vi "test_Checksum U32 - Check Protection with corrupt data.vi"(8 "error in (no error)":errorcluster) -> (0 "error out":errorcluster)   [LabVIEW 2019, in "Protections Unit Tests.lvclass"]
uses:
  Protections Unit Tests.lvclass
  Checksum U32/Checksum U32.lvclass
  0c10e477-a100-4b93-935c-4b2bb0535a3f.vi
  <vilib>/addons/_JKI Toolkits/VI Tester/TestCase.llb/TestCase.lvclass
  C:/Program Files (x86)/National Instruments/LabVIEW 2019/vi.lib/addons/_JKI Toolkits/VI Tester/TestCase.llb/TestCase.lvclass
panel:
  out "Checksum U32 out":refnum<class "Checksum U32.lvclass">
  in  "Checksum U32 in":refnum<class "Checksum U32.lvclass">
  out "TestCase out":refnum<class "Protections Unit Tests.lvclass">
  in  "TestCase in":refnum<class "Protections Unit Tests.lvclass">
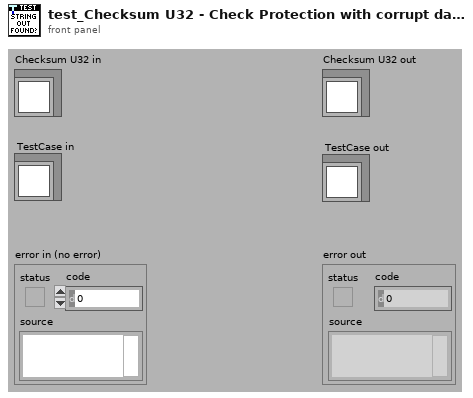
[diagram p1: front panel]
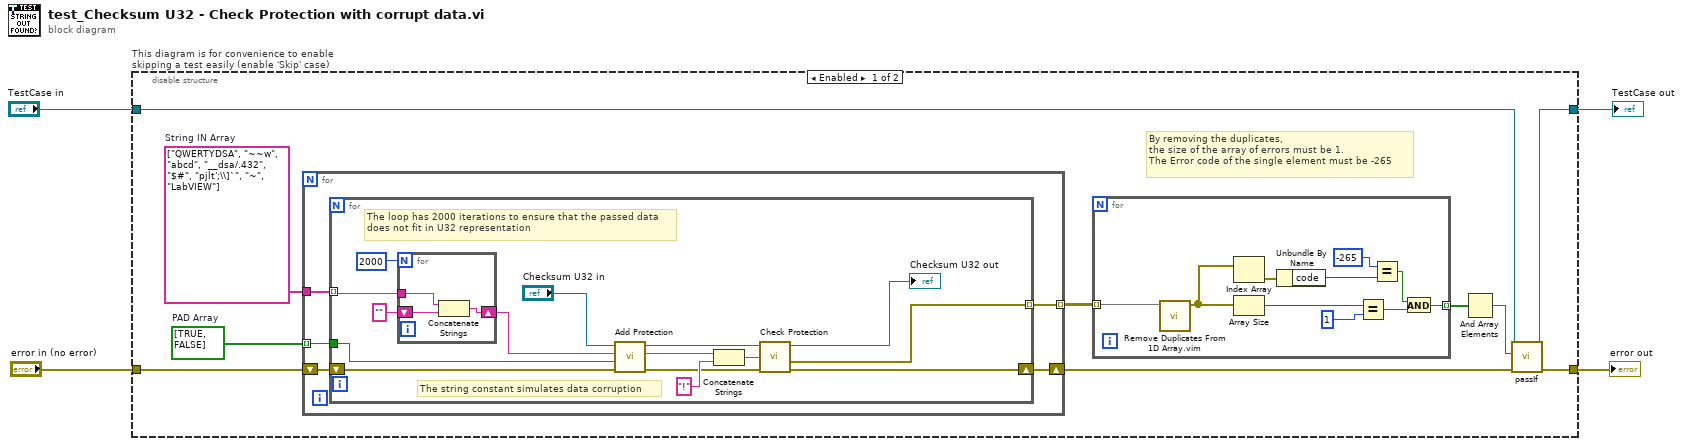
[diagram p0: block diagram]
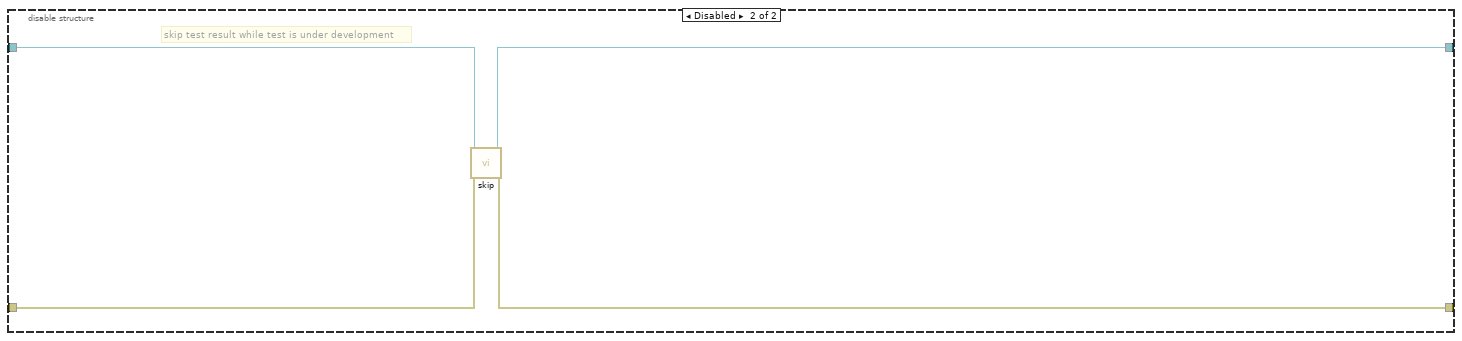
[diagram p2: hidden frame]
diagram:
  n1 = disable-structure "This diagram is for convenience to enable skipping a test easily (enable 'Skip' case)" shown="Enabled" {
    disable-tunnel: "TestCase in" -> [w12 w51]
    disable-tunnel: [w11 w49] -> w1
    disable-tunnel: [w10 w50] -> w3
    disable-tunnel: "error in (no error)" -> [w14 w48]
    frame Enabled {
      w5 = bool[] [TRUE, FALSE]  # PAD Array
      w13 = string[] ["QWERTYDSA", "~~w", "abcd", "__dsa/.432", "$#", "pjlt';\\]`", "~", "LabVIEW"]  # String IN Array
      # "By removing the duplicates, \nthe size of the array of errors must be 1. \nThe Error code of the single element must be -265"
      n2 = for {
        tunnel: w13 -> [w18]
        shift-right: [w17] -> w9
        shift-left: w14 -> [w19]
        tunnel: [w16] -> w6 mode=indexing
        tunnel: w5 -> [w15] mode=indexing
        n3 = for {
          tunnel: w18 -> [w32] mode=indexing
          shift-right: [w27] -> w17
          shift-left: w19 -> [w26]
          tunnel: [w28] -> w16 mode=indexing
          tunnel: w15 -> [w20]
          # "The string constant simulates data corruption"
          # "The loop has 2000 iterations to ensure that the passed data\ndoes not fit in U32 representation"
          n4 = for {
            N: 2000 -> [_]
            shift-right: [w37] -> w25
            shift-left: "" -> [w36]
            tunnel: w32 -> [w35]
            n5 = Concatenate Strings(w35, w36) -> (w37:string)
          }
          n6 = call-dynamic "Add Protection.vi"("error in (no error)"=w26, "Pad"=w20, "String in"=w25, "Checksum U32 in"="Checksum U32 in") -> ("error out"=w24:errorcluster, "String out"=w23:string, "Checksum U32 out"=w22:refnum<class "Checksum U32.lvclass">)  [unwired: 5 in]
          n7 = Concatenate Strings(w23, "!" ("string")) -> (w30:string)
          n8 = call-dynamic "Check Protection.vi"("error in (no error)"=w24, "String in"=w30, "Checksum U32 in"=w22) -> ("error out"=w27:errorcluster, "Protection Error"=w28:errorcluster, "Checksum U32 out"=→"Checksum U32 out":refnum<class "Checksum U32.lvclass">)  [unwired: 5 in, 1 out]
        }
      }
      n9 = for {
        tunnel: w6 -> [w47] mode=indexing
        tunnel: [w42] -> w8 mode=indexing
        n10 = call "Remove Duplicates From 1D Array.vim"("array"=w47) -> ("array with duplicates removed"=w43:errorcluster[])  [unwired: 10 in]
        n11 = Index Array(array=w43) -> (element=w39:errorcluster)  [unwired: 1 in]
        n12 = Array Size(array=w43) -> (size(s)=w38:i32)
        n13 = Unbundle By Name(w39) -> ("code"=w40:i32)
        n14 = Equal?(x=w38, y=1) -> (x = y?=w44:bool)
        n15 = Equal?(x=-265, y=w40) -> (x = y?=w45:bool)
        n16 = And(x=w45, y=w44) -> (x .and. y?=w42:bool)
      }
      n17 = And Array Elements(Boolean array=w8) -> (logical AND=w7:bool)
      n18 = call-dynamic "passIf.vi"("error in (no error)"=w9, "pass"=w7, "TestCase in"=w12) -> ("error out"=w10:errorcluster, "TestCase out"=w11:refnum<class "Protections Unit Tests.lvclass">)  [unwired: 7 in]
    }
    frame Disabled {
      # "skip test result while test is under development"
      n19 = call <vilib>:"skip.vi"("error in (no error)"=w48, "TestCase in"=w51) -> ("error out"=w50:errorcluster, "TestCase out"=w49:refnum<class "Protections Unit Tests.lvclass">)  [unwired: 8 in]
    }
  }
  "error out" <- w3
  "TestCase out" <- w1
